vi "DANTE acquire multiple.vi"(6 "Number of boards in chain":u8(slide)=1 scale=1.0..8.0, 8 "Map points":u32=10, 9 "Time per spectrum [ms]":u32=10 min=1 max=1000000, 10 "Pause button 2":refnum<vi>, 11 "identifier out":string) -> (0 "Statistics":dbl[][](array[numeric]), 1 "spectra":u16[][](array[numeric]), 2 "adv stats":u64[][](array[numeric]))   [LabVIEW 2015]
uses:
  StateTypeDef.ctl
  XGL_DPP.lvlib
panel:
  out "Boards to configure":u8(slide) scale=0.0..8.0
  out "spectra to read 3":i64=10
  out "spectra to read":i64=10
  out "State 2":T1=enum."Close library"
  in  "Add IP":bool
  out "Acq. in progress":bool
  out "Library Initialized":bool
  in  "Get connected":bool
  in  "Init":bool
  in  "Clear":bool
  in  "Close":bool
  in  "Start acq":bool
  in  "Acquisition time [s]":dbl=10.0 min=1.0 max=1000.0
  out "Error code":i32
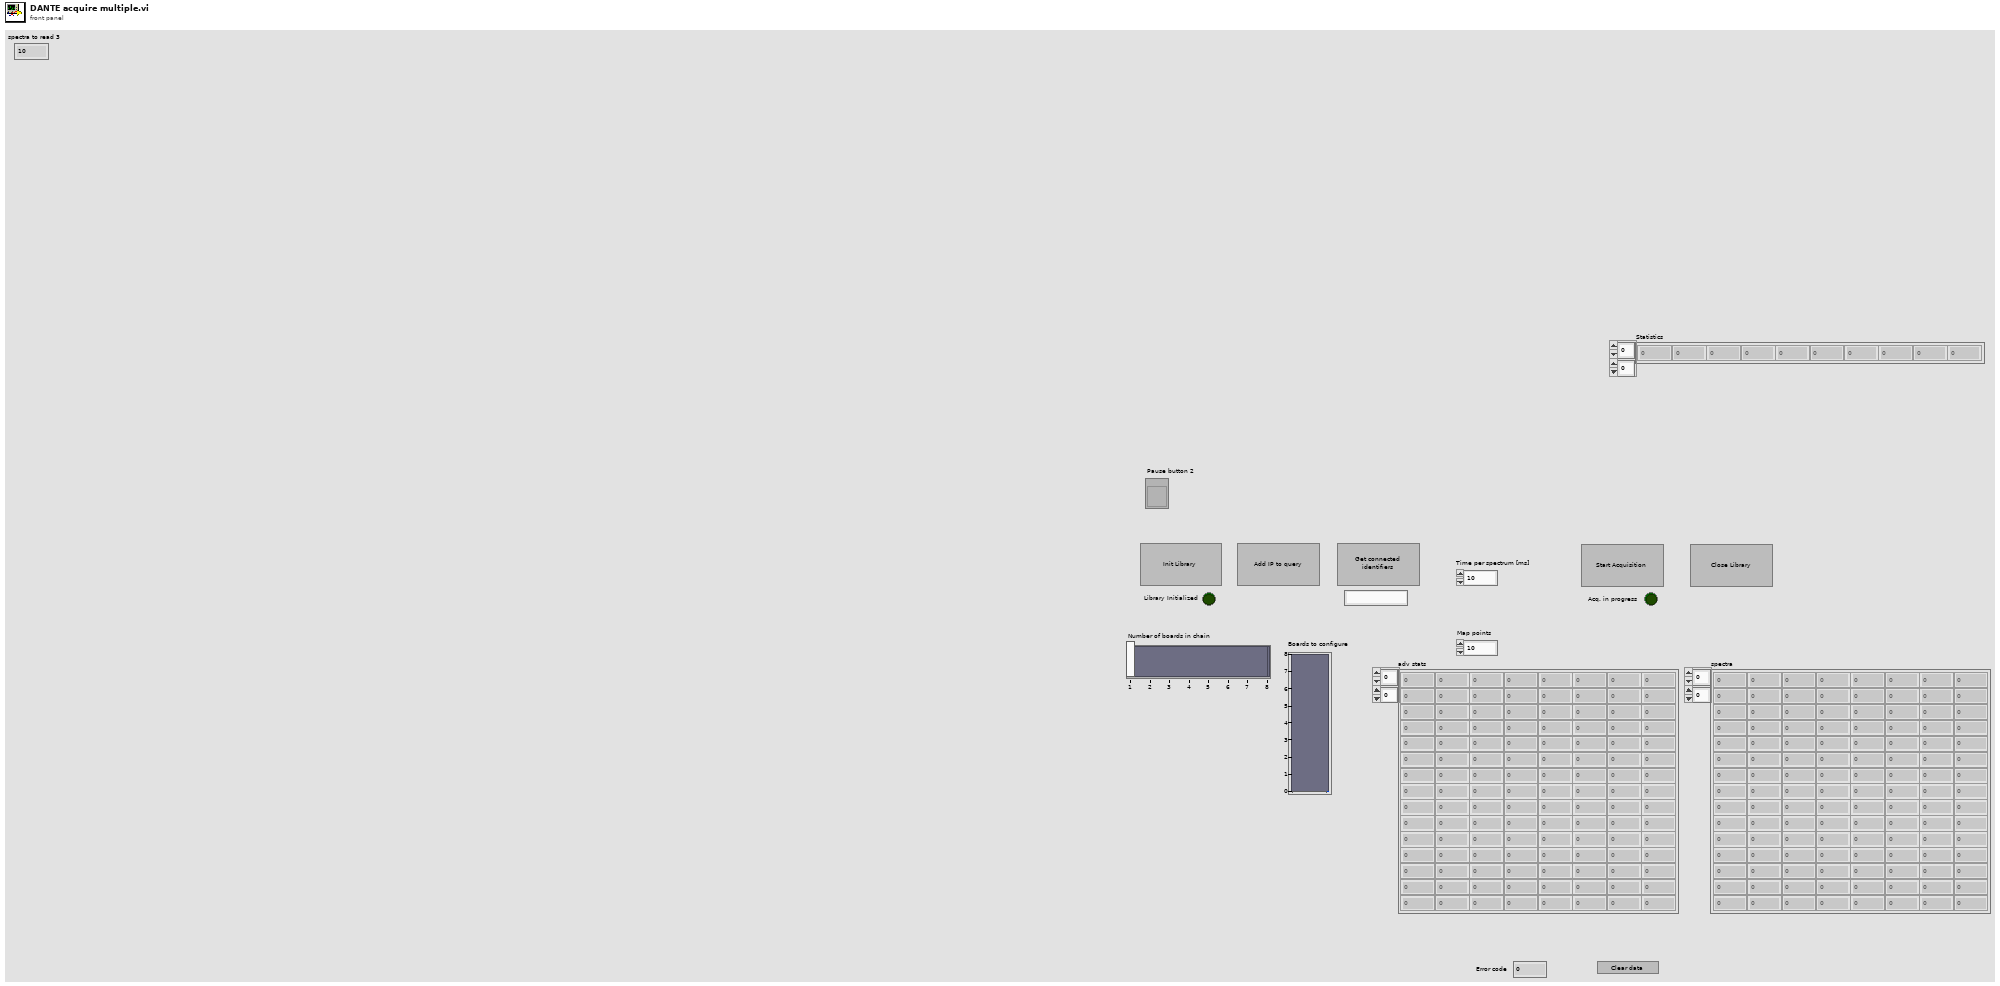
[diagram p1: front panel]
types:
  T1 = typedef "StateTypeDef.ctl" = enum16{"Stop", "Check downloaded spectra", "Get all data", "Read acq mode", "Send running/Get Data", "Add IP to query", "Get serial", "Close library", "Clear", "Acquisition start", "Initialization", "Check Answer", "Configuring", "Wait Answer", "Start map", "Wait input"}
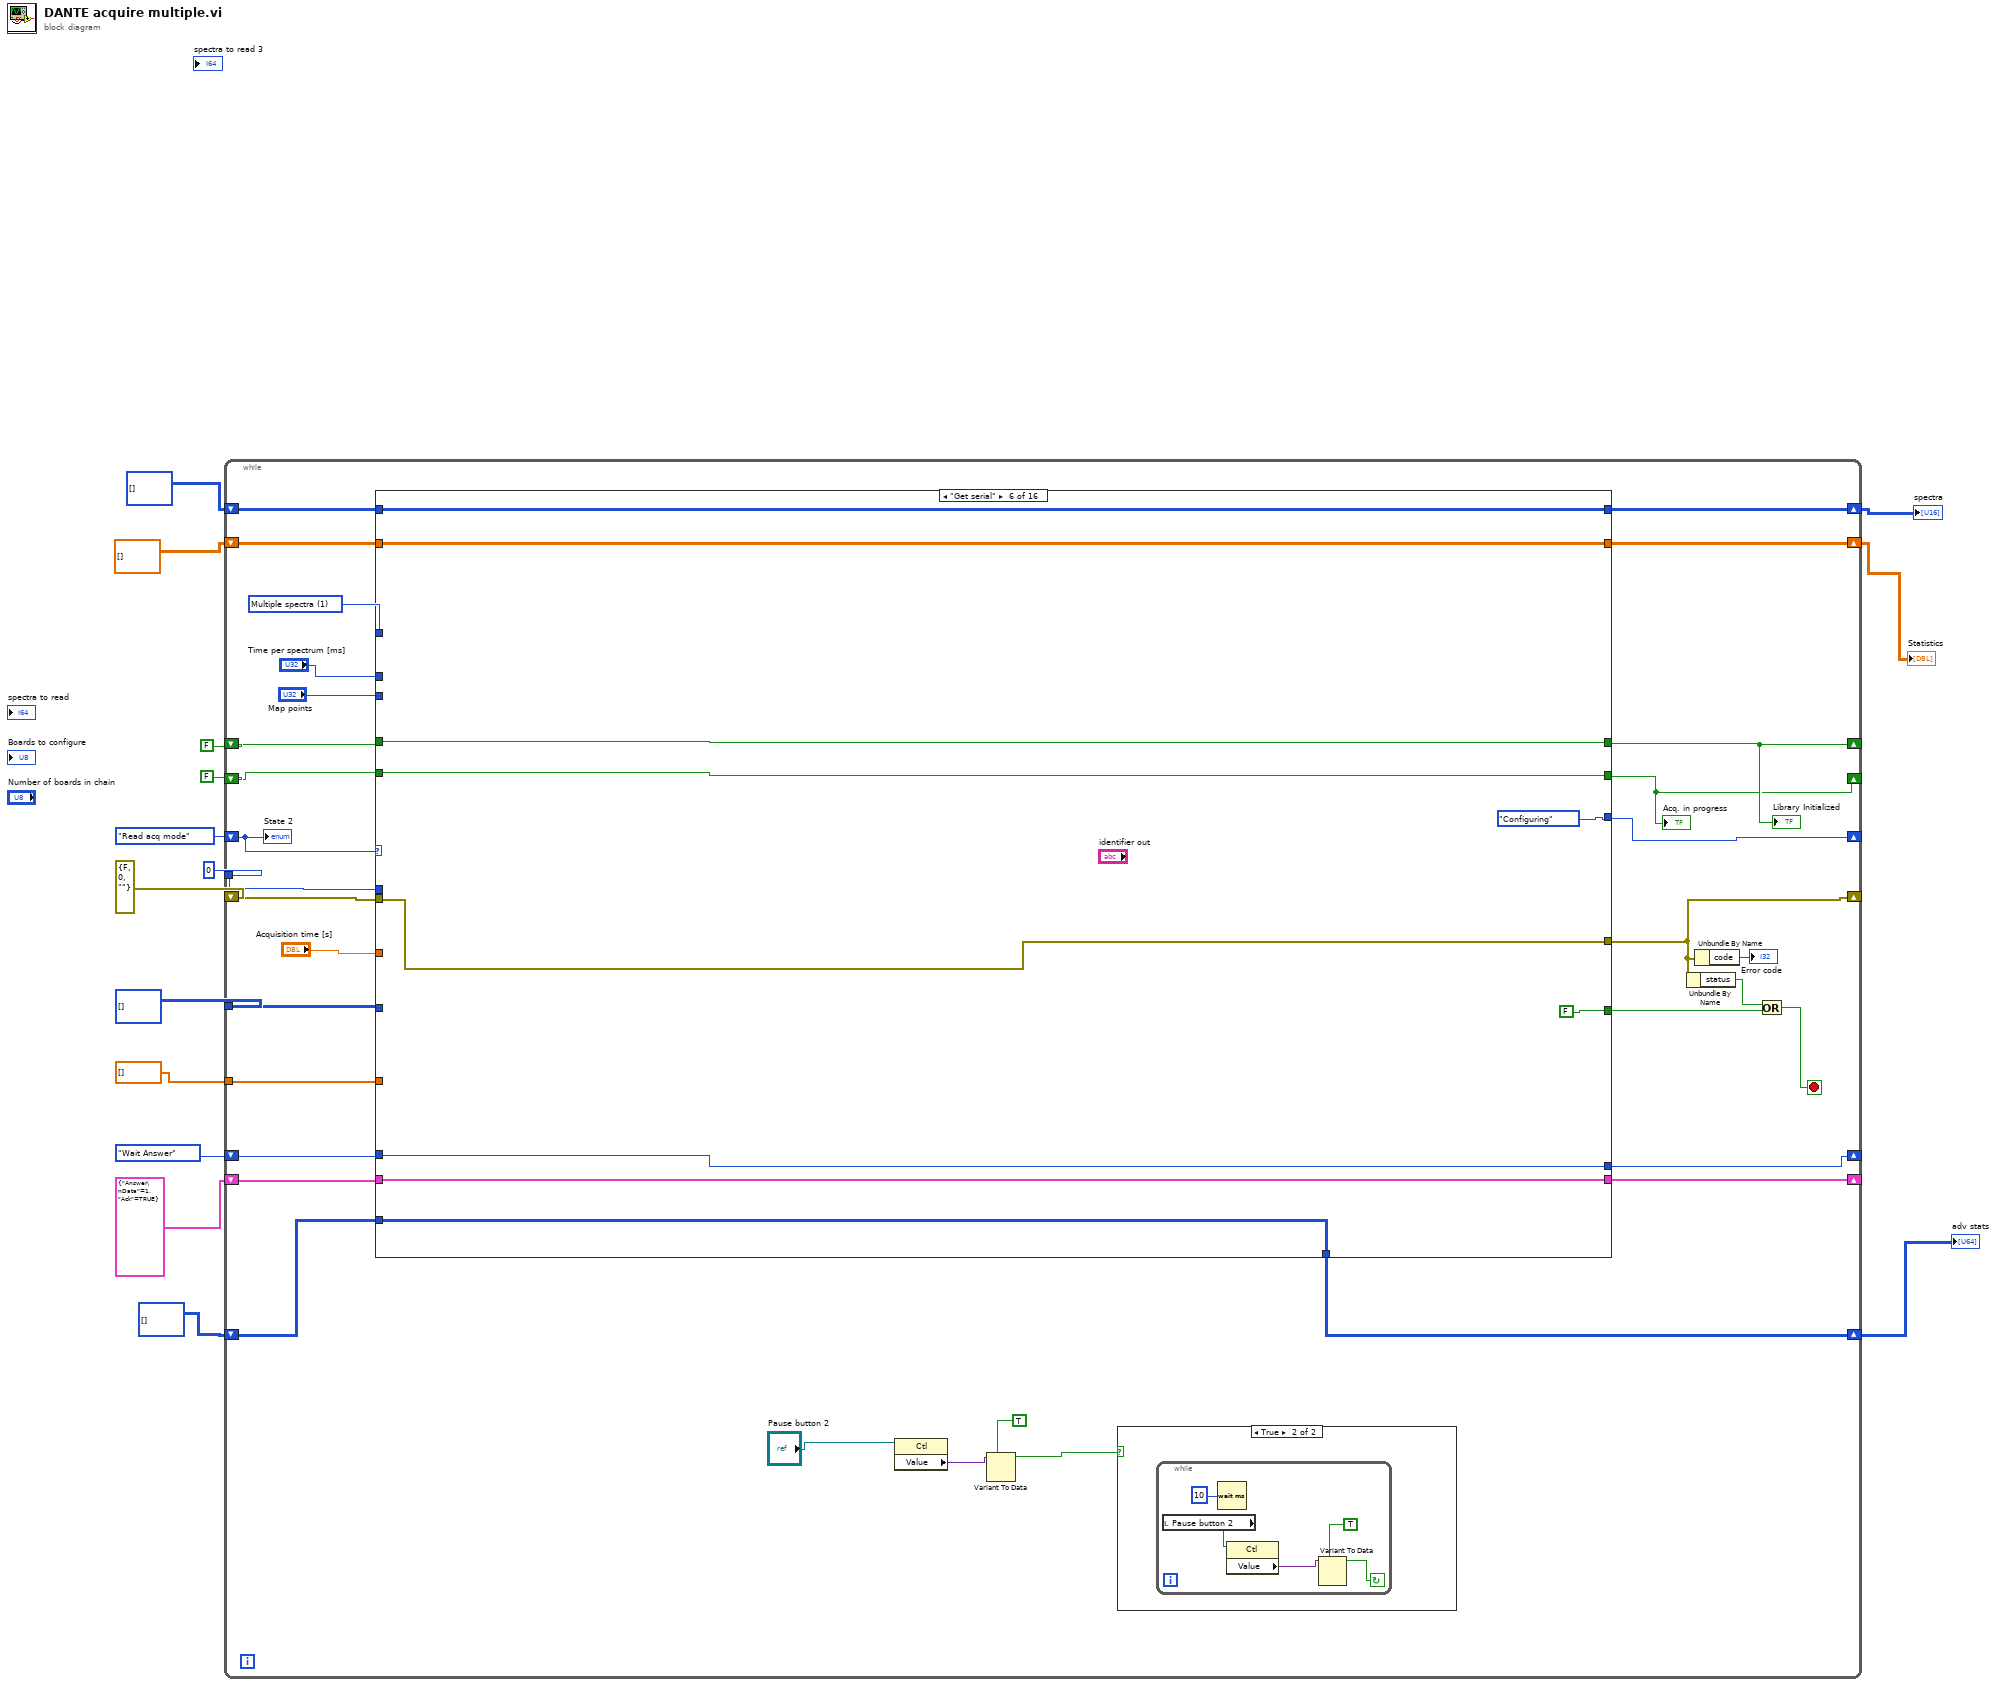
[diagram p0: block diagram]
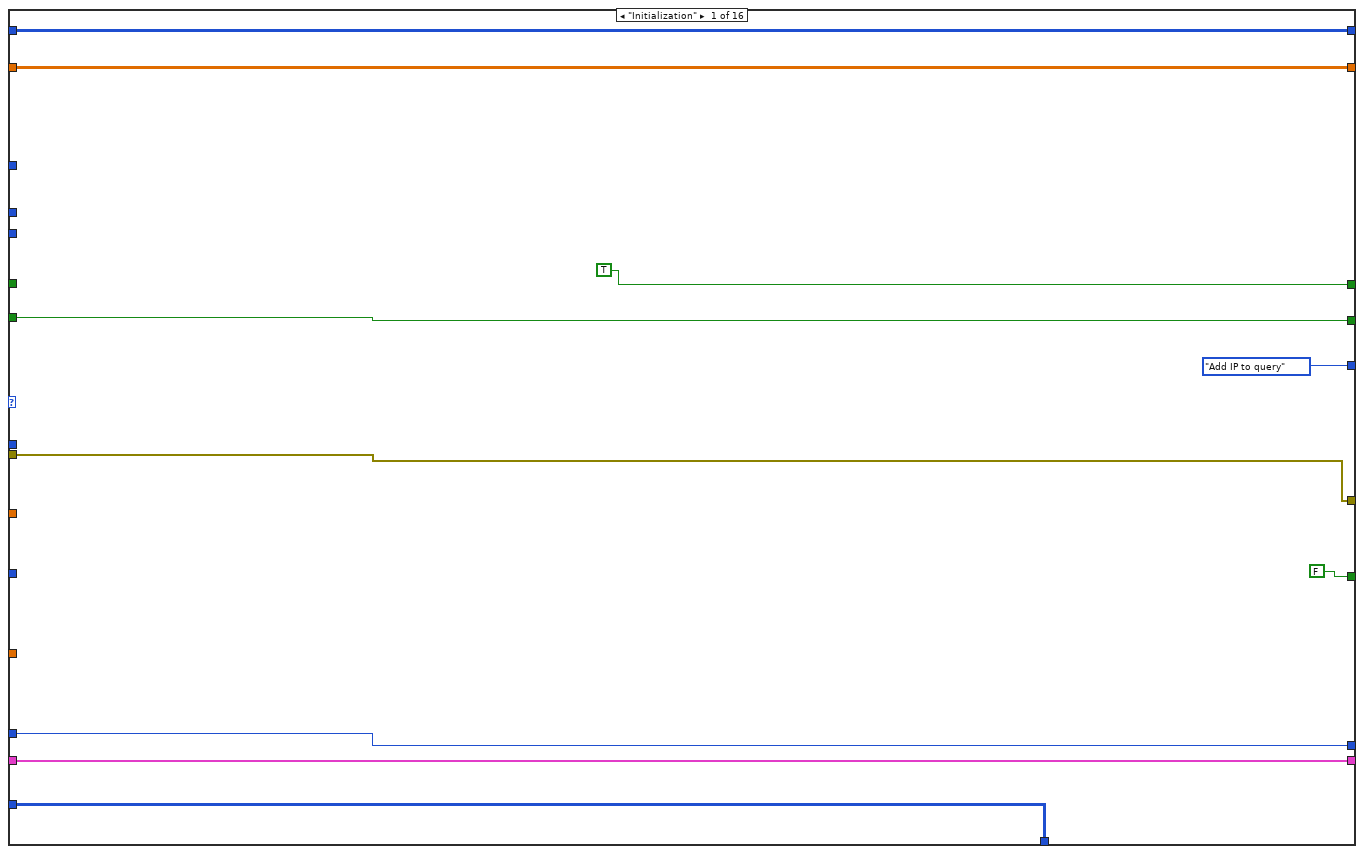
[diagram p3: hidden frame]
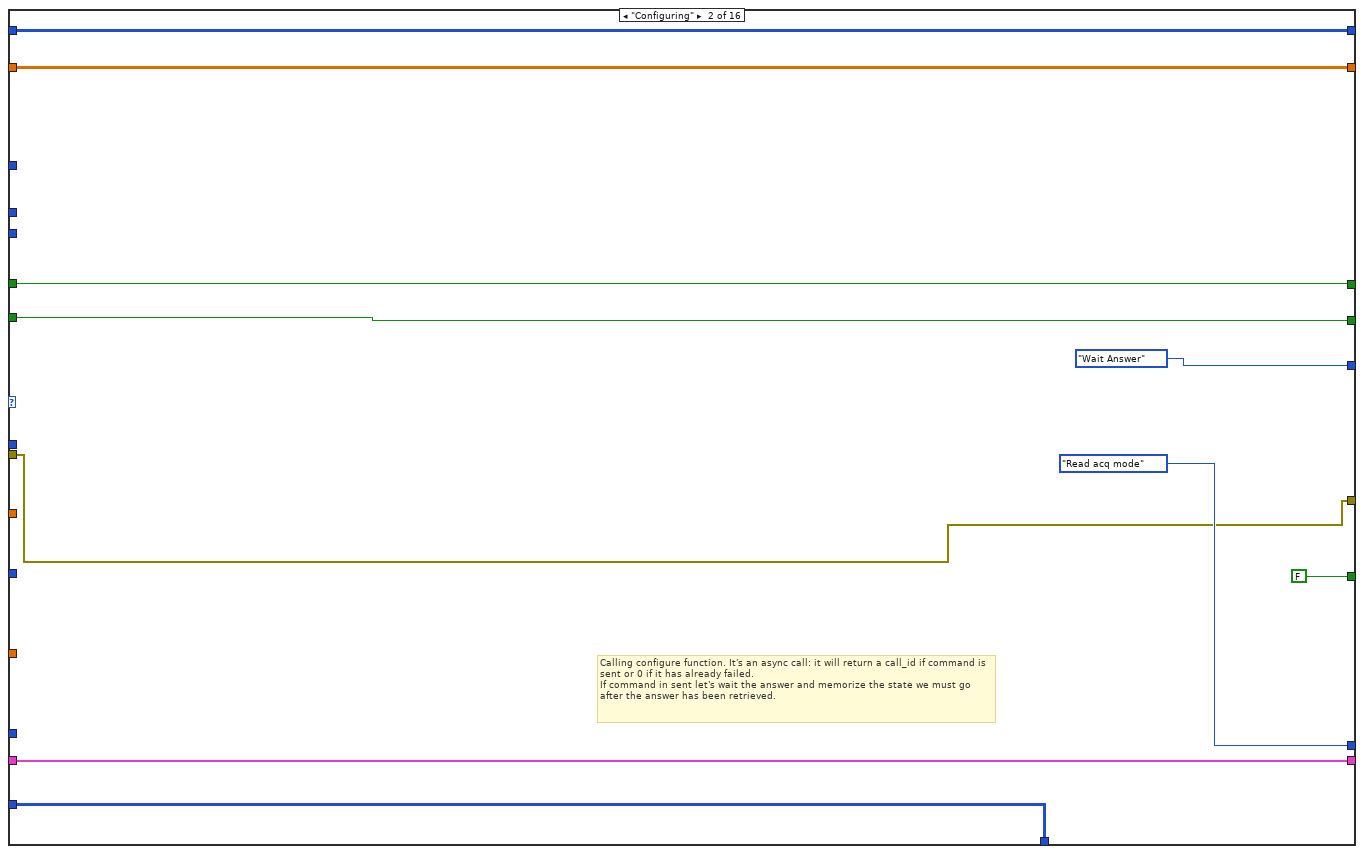
[diagram p4: hidden frame]
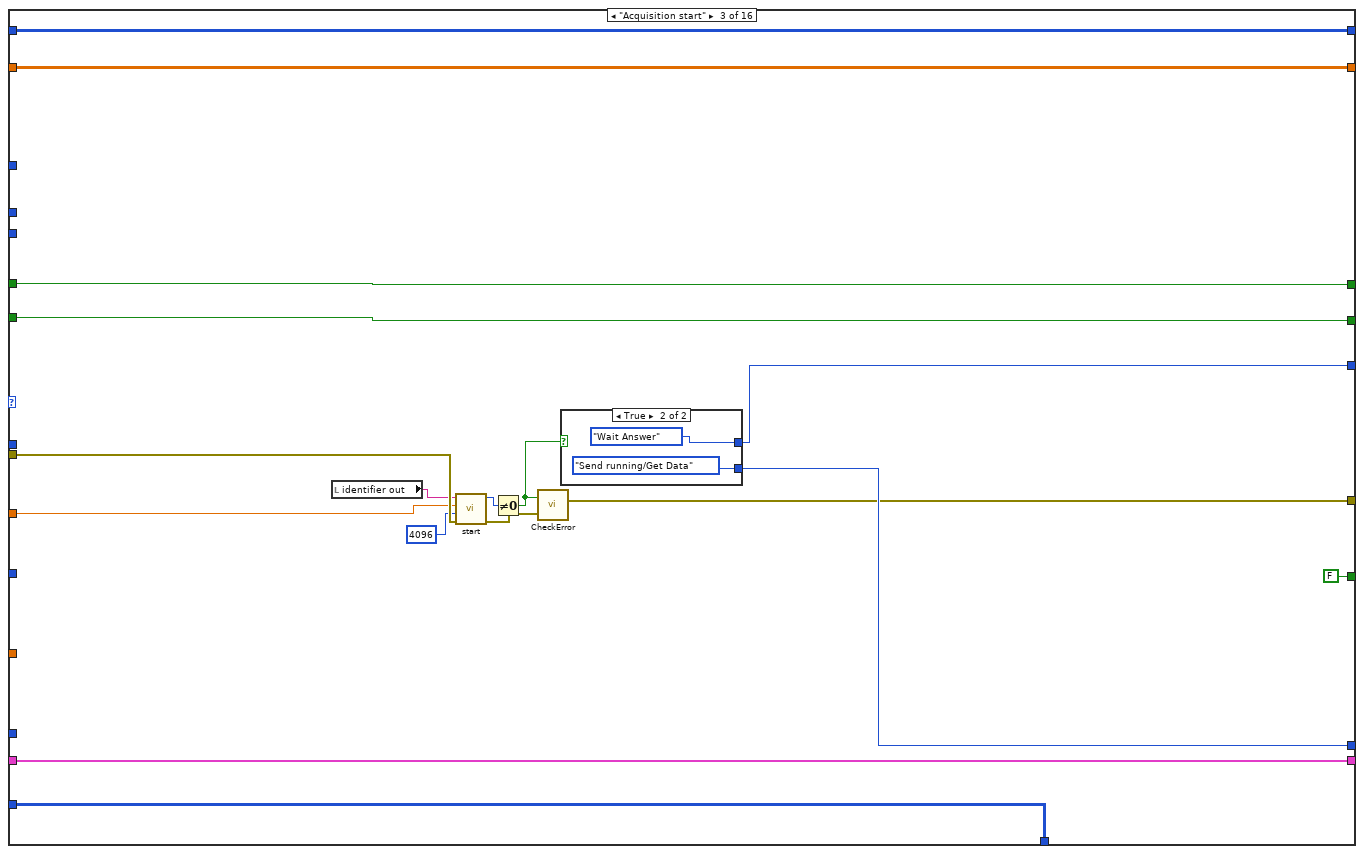
[diagram p5: hidden frame]
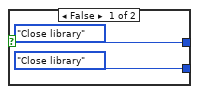
[diagram p6: hidden frame]
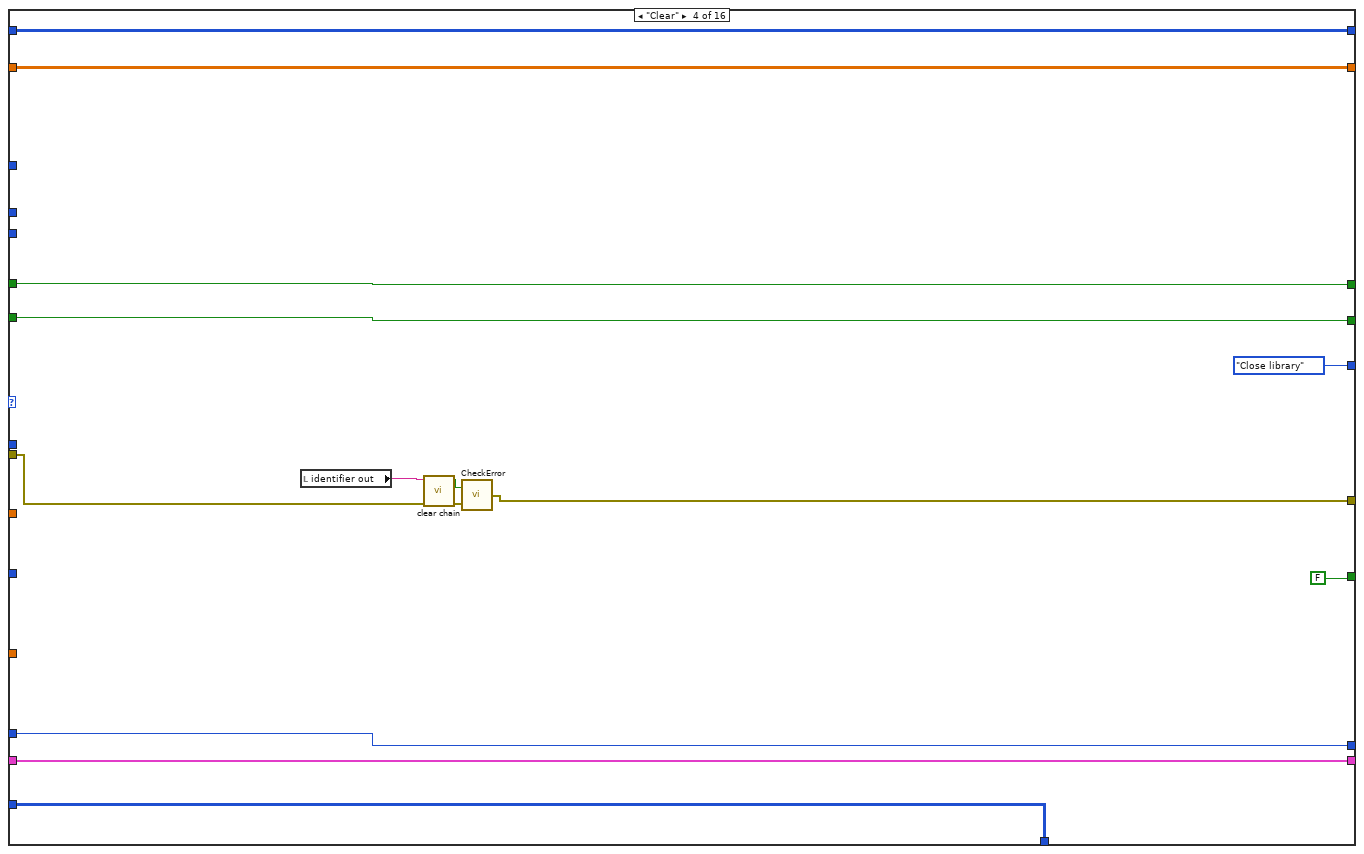
[diagram p7: hidden frame]
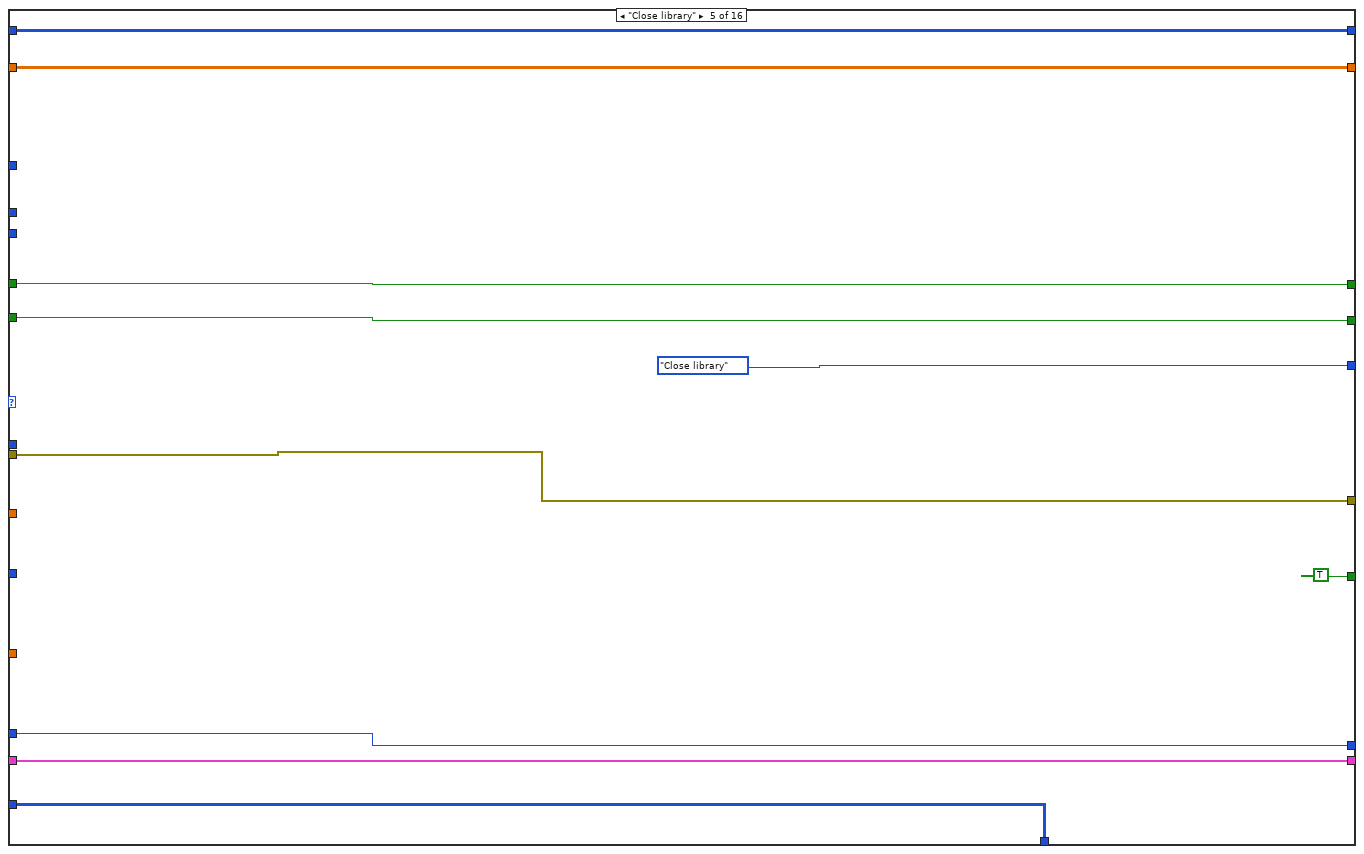
[diagram p8: hidden frame]
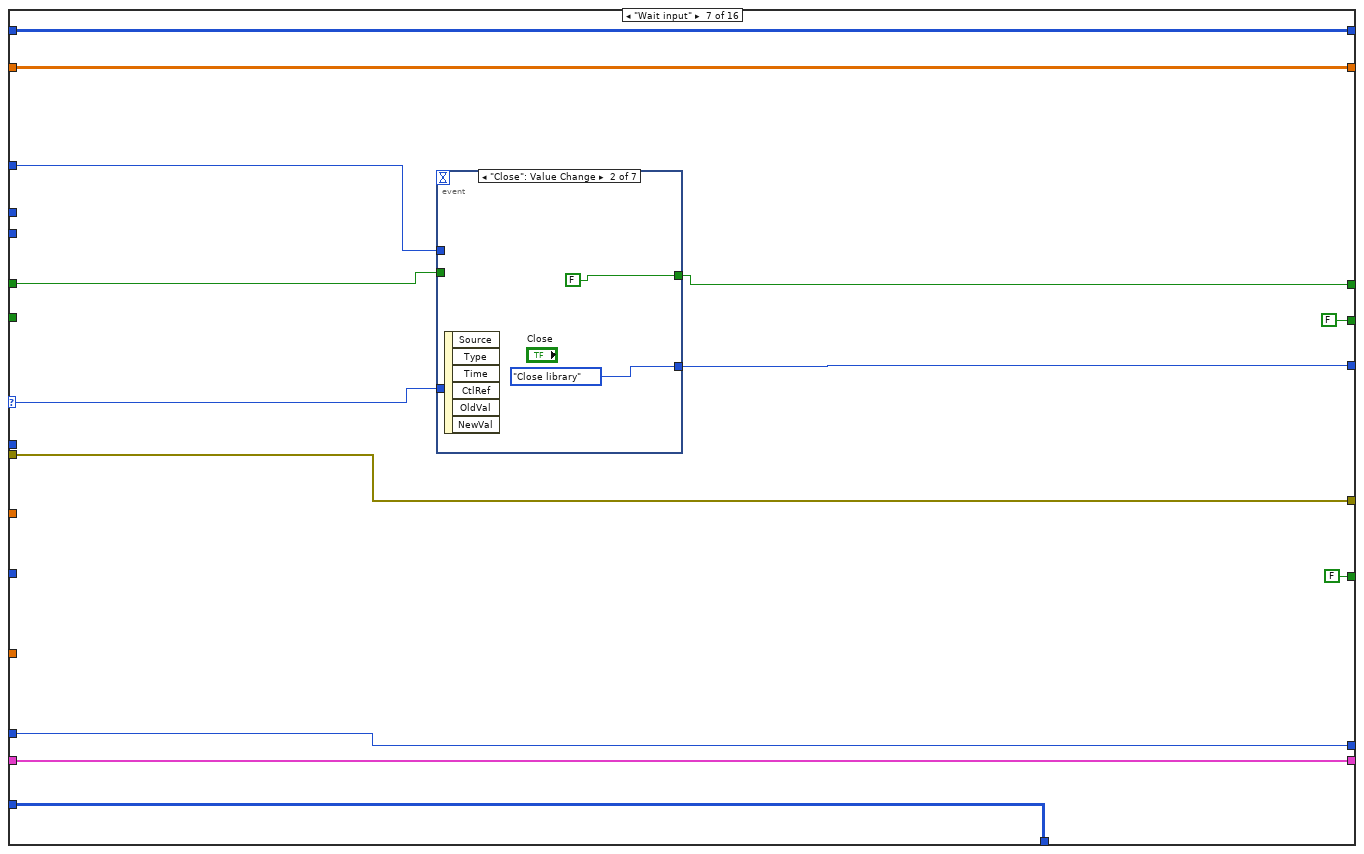
[diagram p9: hidden frame]
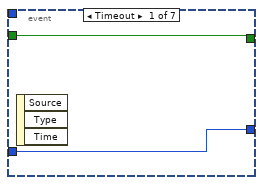
[diagram p10: hidden frame]
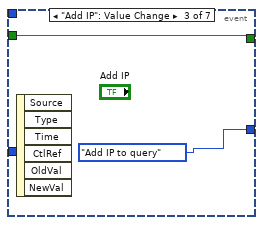
[diagram p11: hidden frame]
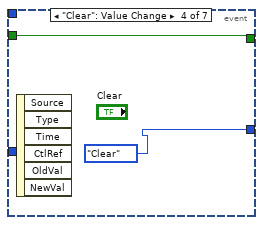
[diagram p12: hidden frame]
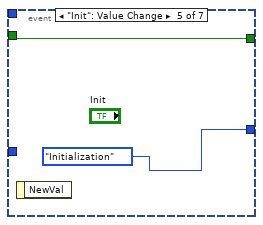
[diagram p13: hidden frame]
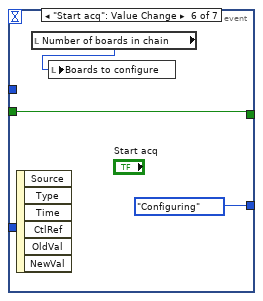
[diagram p14: hidden frame]
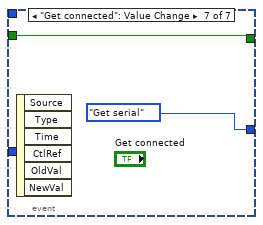
[diagram p15: hidden frame]
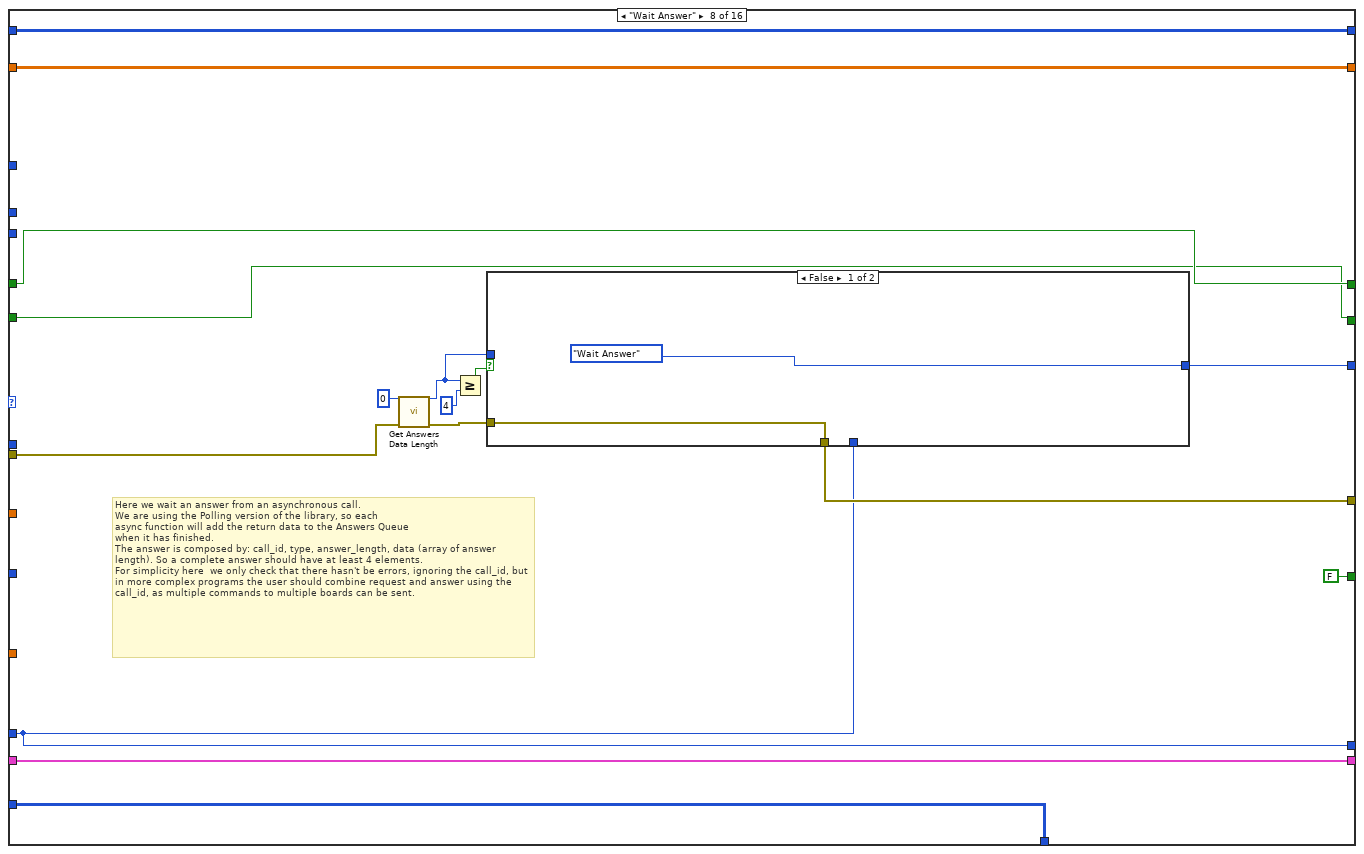
[diagram p16: hidden frame]
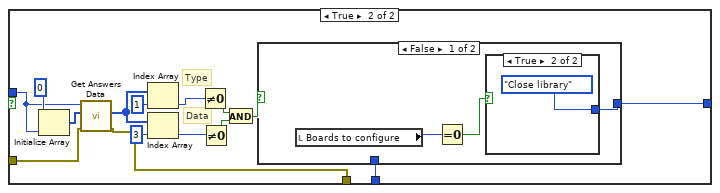
[diagram p17: hidden frame]
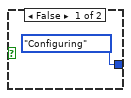
[diagram p18: hidden frame]
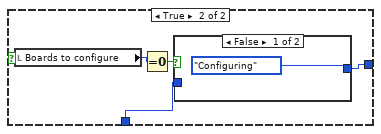
[diagram p19: hidden frame]
diagram:
  n1 = while {
    shift-right: [w46] -> _
    shift-left: errorcluster {"status"=FALSE, "code"=0, "source"=""} ("error in (no error)") -> [w48]
    shift-right: [w34] -> _
    shift-left: StateTypeDef."Read acq mode" ("State") -> [w30]
    shift-right: [w40] -> _
    shift-left: FALSE -> [w41]
    shift-right: [w38] -> _
    shift-left: FALSE -> [w39]
    tunnel: u16 0 ("Board") -> [w37]
    shift-right: [w36] -> _
    shift-left: StateTypeDef."Wait Answer" ("State") -> [w35]
    shift-right: [w32] -> _
    shift-left: cluster{"Answer\nData":i32, "Ack":bool} {"Answer\nData"=1, "Ack"=TRUE} -> [w33]
    tunnel: dbl[] [] ("Y") -> [w27]
    tunnel: u16[][] [] ("element") -> [w26]
    shift-right: [w24] -> w6
    shift-left: u16[][] [] ("spectra") -> [w25]
    shift-right: [w22] -> w3
    shift-left: dbl[][] [] ("spectra") -> [w23]
    shift-right: [w20] -> w1
    shift-left: u16[][] [] ("spectra") -> [w21]
    stop <- w44 stop-if-true
    w31 = u16 1 items=["Single spectrum", "Multiple spectra"] ("Acquisition mode")
    n2 = case shown="\"Get serial\"" w30 {
      selector: w30 -> [_ _ _ _ _ _ w140 _ _ _ _ _ _ _ _ _]
      tunnel: w48 -> [w57 w67 w88 w103 w112 w122 w139 w172 w211 w251 w281 w327 w351 w368 w464 w493]
      tunnel: [w57 w67 w82 w97 w112 w122 w139 w166 w210 w251 w272 w327 w348 w366 w464 w489] -> w46
      tunnel: [StateTypeDef."Add IP to query" ("State") StateTypeDef."Wait Answer" ("State") w86 StateTypeDef."Close library" ("State") StateTypeDef."Close library" ("State") StateTypeDef."Configuring" ("State") w141 w162 w209 StateTypeDef."Get serial" ("State") w266 w330 w347 StateTypeDef."Check downloaded spectra" ("State") w466 StateTypeDef."Wait Answer" ("State")] -> w34
      tunnel: "Acquisition time [s]" -> [_ _ w87 _ _ _ _ _ _ _ _ _ _ _ _ _]
      tunnel: [FALSE ("y") FALSE ("y") FALSE ("y") FALSE ("y") TRUE ("y") FALSE ("y") FALSE ("y") FALSE ("y") FALSE ("y") FALSE ("y") FALSE ("y") FALSE FALSE FALSE FALSE FALSE] -> w42
      tunnel: [TRUE w72 w90 w107 w117 w127 w137 w164 w205 w257 w270 w329 w345 w370 w465 w484] -> w40
      tunnel: w41 -> [_ w72 w90 w107 w117 w127 w136 w164 w205 w257 w270 w329 w345 w370 w465 w484]
      tunnel: [w62 w71 w89 w106 w116 w126 FALSE w163 w204 w256 w264 w328 w344 w371 w453 FALSE] -> w38
      tunnel: w39 -> [w62 w71 w89 w106 w116 w126 _ w163 w204 w256 w263 w328 w344 _ _ _]
      tunnel: w37 -> [_ _ _ _ _ _ _ _ _ _ w282 _ _ _ _ _]
      tunnel: [w61 StateTypeDef."Read acq mode" ("State") w84 w105 w115 w125 w135 w161 w206 w255 w267 w330 w346 w372 w462 StateTypeDef."Get all data" ("State")] -> w36
      tunnel: w35 -> [w61 _ _ w105 w115 w125 w135 w161 w206 w255 _ _ _ w372 w462 _]
      tunnel: w33 -> [w60 w68 w81 w104 w114 w124 w134 w160 w208 w253 w269 w325 w342 w373 w461 w486]
      tunnel: [w60 w68 w81 w104 w114 w124 w134 w160 w207 w253 w268 w325 w342 w373 w461 w486] -> w32
      tunnel: w31 -> [_ _ _ _ _ _ w133 _ _ _ _ w331 _ _ _ _]
      tunnel: "Time per spectrum [ms]" -> [_ _ _ _ _ _ _ _ _ _ _ _ w352 _ w460 _]
      tunnel: "Map points" -> [_ _ _ _ _ _ _ _ _ _ _ _ w339 _ _ _]
      tunnel: w26 -> [_ _ _ _ _ _ _ _ _ _ _ _ _ _ _ _]
      tunnel: w27 -> [_ _ _ _ _ _ _ _ _ _ _ _ _ _ _ _]
      tunnel: w25 -> [w56 w66 w76 w98 w111 w121 w131 w159 w203 w250 w260 w324 w336 w363 w452 w481]
      tunnel: [w56 w66 w76 w98 w111 w121 w131 w159 w203 w250 w260 w324 w336 w362 w452 w481] -> w24
      tunnel: w23 -> [w55 w65 w75 w96 w110 w120 w130 w158 w202 w249 w259 w323 w335 w361 w451 w480]
      tunnel: [w55 w65 w75 w96 w110 w120 w130 w158 w202 w249 w259 w323 w335 w360 w451 w480] -> w22
      tunnel: w21 -> [w54 w64 w74 w95 w109 w119 w129 w157 w201 w248 w258 w322 w334 w359 w450 w479]
      tunnel: [w54 w64 w74 w95 w109 w119 w129 w157 w201 w248 w258 w322 w334 w358 w450 w479] -> w20
      frame "Initialization" {
      }
      frame "Configuring" {
        # "Calling configure function. It's an async call: it will return a call_id if command is sent or 0 if it has already failed.\nIf command in sent let's wait the answer and memorize the state we must go after the answer has been retrieved."
      }
      frame "Acquisition start" {
        n3 = local read "identifier out"() -> (w78:string)
        n4 = call "start.vi"("error in (no error)"=w88, "spect_depth"=u16 4096, "time"=w87, "identifier"=w78) -> ("error out"=w83:errorcluster, "function return"=w80:u32)  [unwired: 6 in]
        n5 = Not Equal To 0?(x=w80) -> (x != 0?=w79:bool)
        n6 = call "CheckError.vi"("error in (no error)"=w83, "ret_val"=w79) -> ("error out"=w82:errorcluster)
        n7 = case shown="True" w79 {
          tunnel: [StateTypeDef."Close library" ("State") StateTypeDef."Wait Answer" ("State")] -> w86
          tunnel: [StateTypeDef."Close library" ("State") StateTypeDef."Send running/Get Data" ("State")] -> w84
          frame False {
          }
          frame True {
          }
        }
      }
      frame "Clear" {
        n8 = local read "identifier out"() -> (w99:string)
        n9 = call "clear chain.vi"("error in (no error)"=w103, "identifier"=w99) -> ("error out"=w101:errorcluster, "function return"=w102:bool)  [unwired: 8 in]
        n10 = call "CheckError.vi"("error in (no error)"=w101, "ret_val"=w102) -> ("error out"=w97:errorcluster)
      }
      frame "Close library" {
      }
      frame "Get serial" {
      }
      frame "Wait input" {
        n11 = event shown="[1] \"Close\": Value Change" {
          selector: _ -> [_ _ _ _ _ _ _]
          dyn-events: _ -> [_ _ _ _ _ _ _]
          timeout: _ -> [_ _ _ _ _ _ _]
          tunnel: [w143 StateTypeDef."Close library" ("State") StateTypeDef."Add IP to query" ("State") StateTypeDef."Clear" ("State") StateTypeDef."Initialization" ("State") StateTypeDef."Configuring" ("State") StateTypeDef."Get serial" ("State")] -> w141
          tunnel: w140 -> [w143 _ _ _ _ _ _]
          tunnel: [w142 FALSE w147 w149 w151 w154 w156] -> w137
          tunnel: w136 -> [w142 _ w147 w149 w151 w154 w156]
          tunnel: w133 -> [_ _ _ _ _ _ _]
          event Timeout {
            n12 = event-data() -> ()  [unwired: 1 in, 3 out]
          }
          event "Close": Value Change {
            n13 = event-data() -> ()  [unwired: 1 in, 6 out]
          }
          event "Add IP": Value Change {
            n14 = event-data() -> ()  [unwired: 1 in, 6 out]
          }
          event "Clear": Value Change {
            n15 = event-data() -> ()  [unwired: 1 in, 6 out]
          }
          event "Init": Value Change {
            n16 = event-data() -> ()  [unwired: 1 in, 1 out]
          }
          event "Start acq": Value Change {
            n17 = event-data() -> ()  [unwired: 1 in, 6 out]
            n18 = local read "Number of boards in chain"() -> (w152:u8)
            n19 = local write "Boards to configure"(w152) -> ()
          }
          event "Get connected": Value Change {
            n20 = event-data() -> ()  [unwired: 1 in, 6 out]
          }
        }
      }
      frame "Wait Answer" {
        # "Here we wait an answer from an asynchronous call.\nWe are using the Polling version of the library, so each\nasync function will add the return data to the Answers Queue\nwhen it has finished.\nThe answer is composed by: call_id, type, answer_length, data (array of answer length). So a complete answer should have at least 4 elements.\nFor simplicity here  we only check that there hasn't be errors, ignoring the call_id, but in more complex programs the user should combine request and answer using the call_id, as multiple commands to multiple boards can be sent."
        n21 = call "Get Answers Data Length.vi"("error in (no error)"=w172, "length"=u32 0) -> ("error out"=w168:errorcluster, "length out"=w167:u32)  [unwired: 7 in, 1 out]
        n22 = Greater Or Equal?(x=w167, y=u32 4) -> (x >= y?=w169:bool)
        n23 = case shown="False" w169 {
          tunnel: w168 -> [w174 w177]
          tunnel: w167 -> [_ w179]
          tunnel: w161 -> [_ w181]
          tunnel: [w174 w176] -> w166
          tunnel: [StateTypeDef."Wait Answer" ("State") w180] -> w162
          frame False {
          }
          frame True {
            # "Data"
            # "Type"
            n24 = Initialize Array(u32 0 ("y"), w179) -> (w178:u32[])
            n25 = call "Get Answers Data.vi"("error in (no error)"=w177, "data"=w178, "length"=w179) -> ("error out"=w176:errorcluster, "data out"=w175:u32[])  [unwired: 4 in, 1 out]
            n26 = Index Array(array=w175, index=1) -> (element=w185:u32)
            n27 = Index Array(array=w175, index=3) -> (element=w186:u32)
            n28 = Not Equal To 0?(x=w185) -> (x != 0?=w183:bool)
            n29 = Not Equal To 0?(x=w186) -> (x != 0?=w184:bool)
            n30 = And(x=w183, y=w184) -> (x .and. y?=w182:bool)
            n31 = case shown="False" w182 {
              tunnel: w181 -> [_ w195]
              tunnel: [w192 w196] -> w180
              frame False {
                n32 = local read "Boards to configure"() -> (w191:u8)
                n33 = Equal To 0?(x=w191) -> (x = 0?=w190:bool)
                n34 = case shown="True" w190 {
                  tunnel: [StateTypeDef."Configuring" ("State") StateTypeDef."Close library" ("State")] -> w192
                  frame False {
                  }
                  frame True {
                  }
                }
              }
              frame True {
                n35 = local read "Boards to configure"() -> (w198:u8)
                n36 = Equal To 0?(x=w198) -> (x = 0?=w197:bool)
                n37 = case shown="False" w197 {
                  tunnel: [StateTypeDef."Configuring" ("State") w200] -> w196
                  tunnel: w195 -> [_ w200]
                  frame False {
                  }
                  frame True {
                  }
                }
              }
            }
          }
        }
      }
      frame "Check Answer" {
        # "Here I check if an answer is available. If it is, I pass the data to a variable.\nThen I return to the 'next state' in any case, even if no answer is yet available."
        n38 = call "Get Answers Data Length.vi"("error in (no error)"=w211, "length"=u32 0) -> ("error out"=w213:errorcluster, "length out"=w212:u32)  [unwired: 7 in, 1 out]
        n39 = Greater Or Equal?(x=w212, y=u32 4) -> (x >= y?=w214:bool)
        n40 = case shown="True" w214 {
          tunnel: w213 -> [w220 w225]
          tunnel: w212 -> [_ w223]
          tunnel: [w220 w231] -> w210
          tunnel: [w219 w230] -> w209
          tunnel: w206 -> [w219 w229]
          tunnel: w208 -> [w218 w227]
          tunnel: [w218 w228] -> w207
          frame False {
            # "Do not update answer data."
          }
          frame True {
            # "Data"
            # "Type"
            n41 = Initialize Array(u32 0 ("y"), w223) -> (w222:u32[])
            n42 = call "Get Answers Data.vi"("error in (no error)"=w225, "data"=w222, "length"=w223) -> ("error out"=w224:errorcluster, "data out"=w221:u32[])  [unwired: 4 in, 1 out]
            n43 = Index Array(array=w221, index=1) -> (element=w233:u32)
            n44 = Index Array(array=w221, index=3) -> (element=w226:u32)
            n45 = Not Equal To 0?(x=w233) -> (x != 0?=w232:bool)
            n46 = case shown="False" w232 {
              selector: w232 -> [w241 w243]
              tunnel: w224 -> [w240 w247]
              tunnel: [w239 w247] -> w231
              tunnel: [StateTypeDef."Close library" ("State") w246] -> w230
              tunnel: w229 -> [_ w246]
              tunnel: [w238 w244] -> w228
              tunnel: w227 -> [w238 w245]
              tunnel: w226 -> [_ w242]
              frame False {
                # "Type = 0, an error occurred."
                n47 = call "CheckError.vi"("error in (no error)"=w240, "ret_val"=w241) -> ("error out"=w239:errorcluster)
              }
              frame True {
                # "Type 1 or 2, which means\nanswer of a read or write cmd."
                n48 = Bundle By Name(cluster=w245, "Answer\nData"=w242, "Ack"=w243) -> (w244:cluster{"Answer\nData":i32, "Ack":bool})
              }
            }
          }
        }
      }
      frame "Add IP to query" {
      }
      frame "Send running/Get Data" {
        w277 = u32 4096 ("spectra_size")
        # "This state basically controls the acquisition. At the beginning the isRunning cmd is sent.\nThe answer will be asynchronous, so we than go to state Check Answer to check only\nonce if the answer is available and we return here.\nIn the meantime we get the data and plot the spectrum as fast as possible.\nThis is one advantage of using asynchrous calls."
        n49 = local read "identifier out"() -> (w262:string)
        n50 = Unbundle By Name(w269) -> ("Ack"=w280:bool)
        n51 = case shown="True" w280 {
          tunnel: w282 -> [w288 w295]
          tunnel: w281 -> [w287 w296]
          tunnel: [w287 w294] -> w273
          tunnel: [w288 w293] -> w271
          tunnel: w269 -> [w286 w298]
          tunnel: [w286 w297] -> w268
          tunnel: [StateTypeDef."Send running/Get Data" ("State") w292] -> w267
          tunnel: [StateTypeDef."Check Answer" ("State") w291] -> w266
          tunnel: [w285 w290] -> w264
          tunnel: w263 -> [w285 _]
          tunnel: w262 -> [_ w289]
          frame False {
            # "Command sent, wait the answer before\nsending another command."
          }
          frame True {
            # "Answer received or cmd not yet sent."
            n52 = Unbundle By Name(w298) -> ("Answer\nData"=w300:i32)
            n53 = Equal To 0?(x=w300) -> (x = 0?=w299:bool)
            n54 = case shown="True" w299 {
              tunnel: [StateTypeDef."Send running/Get Data" ("State") w314] -> w292
              tunnel: [StateTypeDef."Check Answer" ("State") w314] -> w291
              tunnel: w298 -> [w310 w321]
              tunnel: [w309 w318] -> w297
              tunnel: w296 -> [w313 w316]
              tunnel: w295 -> [w307 w317]
              tunnel: [w311 w316] -> w294
              tunnel: [w307 w317] -> w293
              tunnel: [TRUE FALSE] -> w290
              tunnel: w289 -> [w301 _]
              frame False {
                # "Still running."
                n55 = call "is Running system.vi"("error in (no error)"=w313, "Board"=w307, "identifier"=w301) -> ("error out"=w312:errorcluster, "function return"=w304:u32)  [unwired: 7 in]
                n56 = Bundle By Name(cluster=w310, "Ack"=FALSE) -> (w309:cluster{"Answer\nData":i32, "Ack":bool})
                n57 = Not Equal To 0?(x=w304) -> (x != 0?=w305:bool)
                n58 = call "CheckError.vi"("error in (no error)"=w312, "ret_val"=w305) -> ("error out"=w311:errorcluster)
              }
              frame True {
                w314 = StateTypeDef."Close library" ("State")
                # "Board has finished acquisition."
                n59 = Bundle By Name(cluster=w321, "Answer\nData"=1 ("Answer\nData"), "Ack"=TRUE) -> (w318:cluster{"Answer\nData":i32, "Ack":bool})
              }
            }
          }
        }
        n60 = Initialize Array(u64 0 ("acq_status"), w277) -> (w276:u64[])
        n61 = call "get Data.vi"("identifier"=w262, "spectra_size"=w277, "Board"=w271, "id"=u32 0, "values"=w276, "error in (no error)"=w273) -> ("function return"=w274:bool, "values out"=w261:u64[], "error out"=w275:errorcluster)  [unwired: 5 in, 2 out]
        n62 = To Double Precision Float(number=w261) -> ()  [unwired: 1 out]
        n63 = call "CheckError.vi"("error in (no error)"=w275, "ret_val"=w274) -> ("error out"=w272:errorcluster)
      }
      frame "Read acq mode" {
        # "Start issued. Check the selected acquisition mode."
        n64 = case shown="0, Default" w331 {
          tunnel: [StateTypeDef."Acquisition start" ("State") StateTypeDef."Start map" ("State")] -> w330
          frame 0, Default {
          }
          frame 1 {
          }
        }
      }
      frame "Start map" {
        n65 = local read "Number of boards in chain"() -> (w338:u8)
        n66 = local read "identifier out"() -> (w341:string)
        n67 = Multiply(x=w339, y=w338) -> (x*y=w340:u32)
        n68 = local write "spectra to read"(w340) -> ()
        n69 = call "start map.vi"("spect_depth"=u16 4096, "error in (no error)"=w351, "points"=w339, "sp_time"=w352, "identifier"=w341) -> ("error out"=w350:errorcluster, "function return"=w349:u32)  [unwired: 5 in]
        n70 = Not Equal To 0?(x=w349) -> (x != 0?=w353:bool)
        n71 = call "CheckError.vi"("error in (no error)"=w350, "ret_val"=w353) -> ("error out"=w348:errorcluster)
        n72 = case shown="False" w353 {
          tunnel: [StateTypeDef."Close library" ("State") StateTypeDef."Wait Answer" ("State")] -> w347
          tunnel: [StateTypeDef."Close library" ("State") StateTypeDef."Get all data" ("State")] -> w346
          frame False {
          }
          frame True {
          }
        }
      }
      frame "Get all data" {
        # "Get the nb of spectra available and if greater than 0 get them.\nThe spectrum and statistics are returned as 1D arrays (one append to the other)\nso they are reshaped as 2D arrays.\nIn this example all the spectra are stored in a 2D array, that at the end of the measure \nwill have dimensions nb_spectra x 4096. Statistics are just reshaped but not used."
        n73 = local read "Number of boards in chain"() -> (w364:u8)
        n74 = local read "identifier out"() -> (w367:string)
        n75 = for {
          N: w364 -> [_]
          tunnel: [TRUE] -> w371
          tunnel: w367 -> [w386]
          shift-right: [w381] -> w366
          shift-left: w368 -> [w388]
          tunnel: w363 -> [w379]
          tunnel: [w378] -> w362
          tunnel: w361 -> [w377]
          tunnel: [w376] -> w360
          tunnel: w359 -> [w375]
          tunnel: [w374] -> w358
          i -> [w380]
          n76 = call "get Available Data.vi"("error in (no error)"=w388, "Board"=w380, "identifier"=w386) -> ("error out"=w403:errorcluster, "data_number out"=w389:u32, "function return"=w404:bool)  [unwired: 6 in]
          n77 = Greater Than 0?(x=w389) -> (x > 0?=w402:bool)
          n78 = call "CheckError.vi"("error in (no error)"=w403, "ret_val"=w404) -> ("error out"=w401:errorcluster)
          n79 = Multiply(x=w389, y=u32 4096) -> (x*y=w396:u32)
          n80 = Multiply(x=w389, y=u32 4) -> (x*y=w393:u32)
          n81 = Multiply(x=w389, y=u32 24) -> (x*y=w390:u32)
          n82 = Initialize Array(u32 0, w389) -> (w387:u32[])
          n83 = Initialize Array(u16 0, w396) -> (w385:u16[])
          n84 = Initialize Array(0.0, w393) -> (w384:dbl[])
          n85 = Initialize Array(u64 0, w390) -> (w383:u64[])
          n86 = case shown="True" w402 {
            tunnel: w380 -> [_ w434]
            tunnel: w401 -> [w408 w431]
            tunnel: [w408 w444] -> w381
            tunnel: w386 -> [_ w440]
            tunnel: w389 -> [_ w427]
            tunnel: w387 -> [_ w433]
            tunnel: w385 -> [_ w432]
            tunnel: u32 4096 ("spectra_size") -> [_ w430]
            tunnel: w384 -> [_ w429]
            tunnel: w383 -> [_ w428]
            tunnel: w380 -> [_ _]
            tunnel: w379 -> [w407 w423]
            tunnel: [w407 w421] -> w378
            tunnel: w377 -> [w406 w417]
            tunnel: [w406 w416] -> w376
            tunnel: w375 -> [w405 w414]
            tunnel: [w405 w410] -> w374
            frame False {
              # "No spectrum available."
            }
            frame True {
              # "Adv stats reshaped"
              # "Statistics reshaped"
              # "Spectra reshaped"
              n87 = call "get All Data.vi"("identifier"=w440, "data_number"=w427, "id"=w433, "values"=w432, "error in (no error)"=w431, "spectra_size"=w430, "Board"=w434, "stats"=w429, "advstats"=w428) -> ("advstats out"=w447:u64[], "stats out"=w448:dbl[], "function return"=w446:bool, "values out"=w449:u16[], "error out"=w445:errorcluster)  [unwired: 3 in, 3 out]
              n88 = call "CheckError.vi"("error in (no error)"=w445, "ret_val"=w446) -> ("error out"=w444:errorcluster)
              n89 = Reshape Array(w447, w427, 11 ("dimension size")) -> (w409:u64[][])
              n90 = Reshape Array(w448, w427, 4 ("dimension size")) -> (w415:dbl[][])
              n91 = Reshape Array(w449, w427, u16 4096 ("dimension size")) -> (w422:u16[][])
              n92 = Array Size(array=w414) -> (size(s)=w413:i32[])
              n93 = Index Array(array=w413, index=0) -> (element=w411:i32)
              n94 = Insert Into Array(array=w414, index (row)=w411, new element=w409) -> (w410:u16[][])  [unwired: 1 in]
              n95 = local read "spectra to read"() -> (w437:i64)
              n96 = Array Size(array=w422) -> (size(s)=w439:i32[])
              n97 = Array Size(array=w423) -> (size(s)=w424:i32[])
              n98 = Array Size(array=w417) -> (size(s)=w420:i32[])
              n99 = Index Array(array=w439, index=0) -> (element=w436:i32)
              n100 = Index Array(array=w424, index=0) -> (element=w426:i32)
              n101 = Subtract(x=w437, y=w436) -> (x-y=w435:i64)
              n102 = Index Array(array=w420, index=0) -> (element=w418:i32)
              n103 = local write "spectra to read"(w435) -> ()
              n104 = Insert Into Array(array=w423, index (row)=w426, new element=w422) -> (w421:u16[][])  [unwired: 1 in]
              n105 = Insert Into Array(array=w417, index (row)=w418, new element=w415) -> (w416:dbl[][])  [unwired: 1 in]
            }
          }
        }
      }
      frame "Check downloaded spectra" {
        # "Check the current dimension of spectra 2D array. There can be this cases:\n- Downloaded spectra less than total_spectra-1 -> acquisition still in progress.\n- Down spectra equals total_spectra-1 ->acquisition almost finished, send stop.\nNote that the last spectrum will become available after the stop is sent. This because\nthe DLL mark as complete a spectrum if another spectrum arrives or the stop is issued.\n- Down spectra equals total_spectra -> acquisition finished, return to Wait Input."
        n106 = local read "Number of boards in chain"() -> (w454:u8)
        n107 = local read "spectra to read"() -> (w456:i64)
        n108 = Divide(x=w456, y=w454) -> (x/y=w455:dbl)
        n109 = Decrement(x=w455) -> (x-1=w459:dbl)
        n110 = Less Or Equal?(x=w459, y=u32 0) -> (x <= y?=w457:bool)
        n111 = case shown="True" w457 {
          tunnel: [StateTypeDef."Get all data" ("State") w473] -> w466
          tunnel: w460 -> [_ w472]
          tunnel: w459 -> [_ w471]
          tunnel: [TRUE w469] -> w453
          frame False {
          }
          frame True {
            n112 = Equal To 0?(x=w471) -> (x = 0?=w470:bool)
            n113 = case shown="False" w470 {
              tunnel: [StateTypeDef."Stop" ("State") StateTypeDef."Close library" ("State")] -> w473
              tunnel: w472 -> [w475 _]
              tunnel: [TRUE FALSE] -> w469
              frame True {
                n114 = Wait (ms)(milliseconds to wait=w475) -> ()  [unwired: 1 out]
              }
              frame False {
              }
            }
          }
        }
      }
      frame "Stop" {
        n115 = local read "identifier out"() -> (w482:string)
        n116 = call "stop.vi"("error in (no error)"=w493, "identifier"=w482) -> ("error out"=w490:errorcluster, "function return"=w492:u32)  [unwired: 8 in]
        n117 = Not Equal To 0?(x=w492) -> (x != 0?=w491:bool)
        n118 = call "CheckError.vi"("error in (no error)"=w490, "ret_val"=w491) -> ("error out"=w489:errorcluster)
      }
    }
    "Library Initialized" <- w40
    "Acq. in progress" <- w38
    n119 = property on="Property Node" class="Ctl"(reference="Pause button 2") -> ("Value"=w19:variant)  [unwired: 1 in, 2 out]
    n120 = Variant To Data(type=TRUE, Variant=w19) -> (data=w16:bool)  [unwired: 1 in, 1 out]
    n121 = case shown="True" w16 {
      frame False {
      }
      frame True {
        n122 = while {
          stop <- w49 continue-if-true
          n123 = local read "Pause button 2"() -> (w50:refnum<vi>)
          n124 = Wait (ms)(milliseconds to wait=u32 10) -> ()  [unwired: 1 out]
          n125 = property on="Property Node" class="Ctl"(reference=w50) -> ("Value"=w52:variant)  [unwired: 1 in, 2 out]
          n126 = Variant To Data(type=TRUE, Variant=w52) -> (data=w49:bool)  [unwired: 1 in, 1 out]
        }
      }
    }
    n127 = Unbundle By Name(w46) -> ("status"=w43:bool)
    n128 = Unbundle By Name(w46) -> ("code"=→"Error code":i32)
    n129 = Or(x=w43, y=w42) -> (x .or. y?=w44:bool)
    "State 2" <- w30
  }
  "spectra" <- w6
  "Statistics" <- w3
  "adv stats" <- w1
